vi "AWG Waveform Generator.vi"() -> ()   [LabVIEW 2020]
doc: "This example shows how to use the Arbitrary Waveform mode."
uses:
  <instrlib>/niFgen/niFgen.llb/niFgen Output Mode.ctl
  <instrlib>/niFgen/niFgen.llb/niFgen Trigger Mode.ctl
  <instrlib>/niFgen/niFgen.llb/niFgen Create Waveform (WDT).vi
panel:
  in  "Transient":T1={"t1 (ms)"=10.0, "t2 (ms)"=10.0, "t3 (ms)"=10.0, "High Load (A)"=1.0, "Low Load (A)"=0.0, "Slew rate A/us"=0.001}
  in  "error out":errorcluster
  out "Max Waveform size-Read":i32 format="%_1p"
  out "Waveform Graph":waveform(dbl)(graph)
  in  "Update":bool
  in  "DC Offset (V)":dbl(knob) scale=-0.5..0.5 scale format="%#.1f"
  in  "Gain":dbl(knob)=1.0 min=0.0 max=5.0 scale=0.0..10.0 scale format="%#.1f"
  in  "Stop":bool
  in  "FGEN Resource Name":refnum<k15>
  out "Actual Sample Rate (S/s)":dbl format="%.2p"
  in  "Sample Rate (S/s)":dbl=20000000.0 format="%.2p"
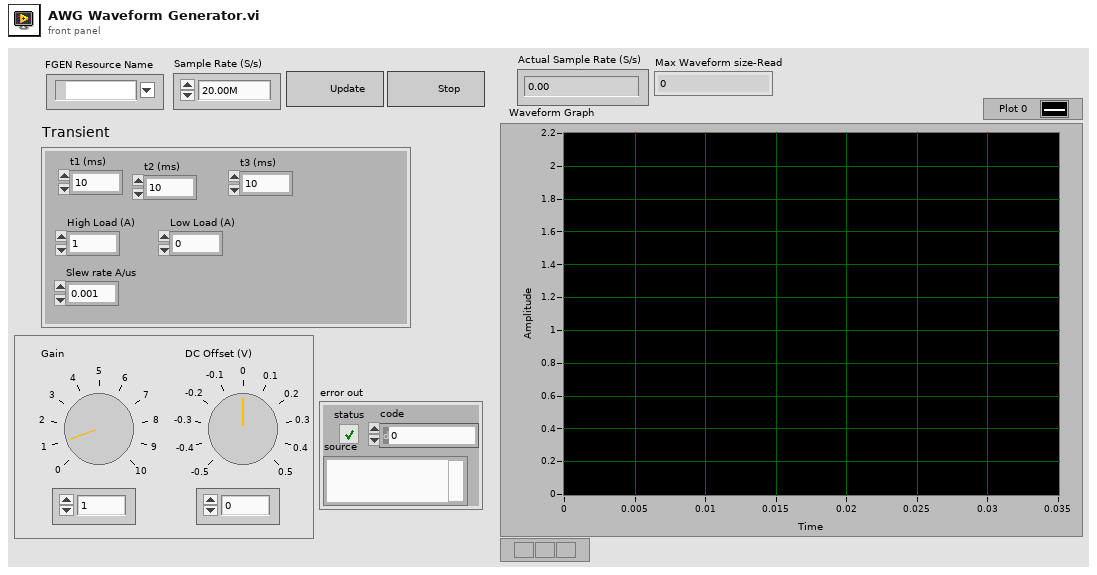
[diagram p1: front panel]
types:
  T1 = cluster{"t1 (ms)":dbl, "t2 (ms)":dbl, "t3 (ms)":dbl, "High Load (A)":dbl, "Low Load (A)":dbl, "Slew rate A/us":dbl}
  T2 = typedef "niFgen Trigger Mode.ctl" = i32
  T3 = typedef "niFgen Output Mode.ctl" = u32
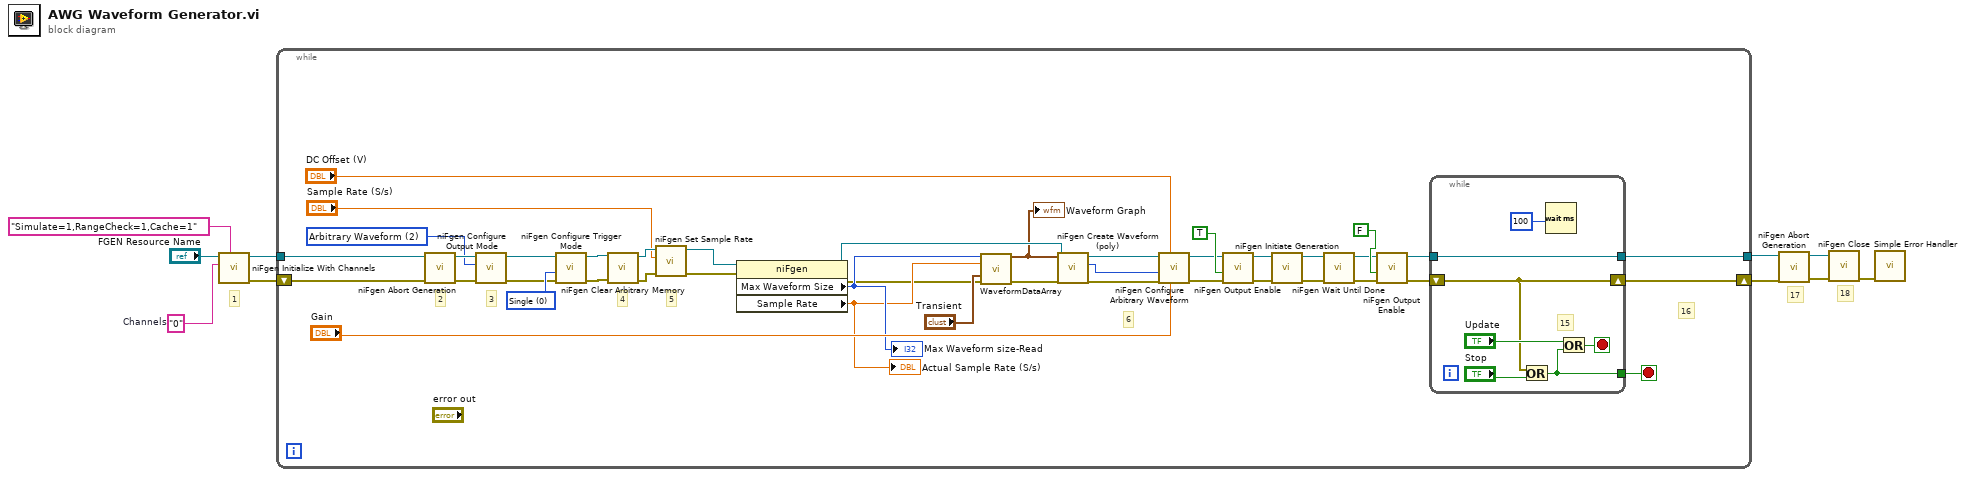
[diagram p0: block diagram]
diagram:
  w4 = "0"  # Channels
  # "18"
  # "17"
  # "1"
  n1 = call <instrlib>:"niFgen Initialize With Channels.vi"("Option String"="Simulate=1,RangeCheck=1,Cache=1", "Channel Name"=w4, "Resource Name"="FGEN Resource Name") -> ("error out"=w3:errorcluster, "Instrument Handle Out"=w2:refnum<k15>)  [unwired: 7 in]
  n2 = while {
    tunnel: [w11] -> w10
    tunnel: w2 -> [w51]
    shift-right: [w13] -> w6
    shift-left: w3 -> [w42]
    stop <- w39 stop-if-true
    w29 = T2 0 items=["Single", "Continuous", "Stepped", "Burst"] ("Trigger Mode")
    w44 = T3 2 items=["Standard Function", "Frequency List", "Arbitrary Waveform", "Arbitrary Sequence", "Script"] ("Output Mode")
    # "16"
    # "6"
    # "5"
    # "4"
    # "3"
    # "2"
    n3 = call <instrlib>:"niFgen Abort Generation.vi"("error in (no error)"=w42, "Instrument Handle"=w51) -> ("error out"=w48:errorcluster, "Instrument Handle Out"=w47:refnum<k15>)  [unwired: 8 in]
    n4 = call <instrlib>:"niFgen Configure Output Mode.vi"("error in (no error)"=w48, "Output Mode (default: 0=Standard Function)"=w44, "Instrument Handle"=w47) -> ("error out"=w27:errorcluster, "Instrument Handle Out"=w28:refnum<k15>)  [unwired: 6 in]
    n5 = call <instrlib>:"niFgen Configure Trigger Mode.vi"("error in (no error)"=w27, "Trigger Mode (default: 1=continuous)"=w29, "Instrument Handle"=w28) -> ("error out"=w25:errorcluster, "Instrument Handle Out"=w26:refnum<k15>)  [unwired: 7 in]
    n6 = call <instrlib>:"niFgen Clear Arbitrary Memory.vi"("error in (no error)"=w25, "Instrument Handle"=w26) -> ("error out"=w35:errorcluster, "Instrument Handle Out"=w36:refnum<k15>)  [unwired: 8 in]
    n7 = call <instrlib>:"niFgen Set Sample Rate.vi"("error in (no error)"=w35, "Sample Rate (Samp/s)"="Sample Rate (S/s)", "Instrument Handle"=w36) -> ("error out"=w30:errorcluster, "Instrument Handle Out"=w31:refnum<k15>)  [unwired: 7 in]
    n8 = property class="niFgen"(reference=w31, error in=w30) -> (reference out=w19:refnum<k15>, error out=w21:errorcluster, "Max Waveform Size"=w23:i32, "Sample Rate"=w22:dbl)
    "Actual Sample Rate (S/s)" <- w22
    "Max Waveform size-Read" <- w23
    n9 = call "WaveformDataArray.vi"("Max Waveform Size"=w23, "Sample Rate"=w22, "Transient"="Transient", "error in"=w21) -> ("Waveform Graph 2"=w18:waveform(dbl), "error out"=w20:errorcluster)  [unwired: 9 in, 1 out]
    "Waveform Graph" <- w18
    n10 = call-poly <instrlib>:"niFgen Create Waveform (poly).vi"("error in (no error)"=w20, "Waveform"=w18, "Instrument Handle"=w19) -> ("error out"=w49:errorcluster, "Waveform Handle"=w37:i32, "Instrument Handle Out"=w50:refnum<k15>)  [unwired: 6 in]
    n11 = call <instrlib>:"niFgen Configure Arbitrary Waveform.vi"("Gain"="Gain", "Offset"="DC Offset (V)", "error in (no error)"=w49, "Waveform Handle"=w37, "Instrument Handle"=w50) -> ("error out"=w32:errorcluster, "Instrument Handle Out"=w33:refnum<k15>)  [unwired: 5 in]
    n12 = call <instrlib>:"niFgen Output Enable.vi"("error in (no error)"=w32, "Output Enable (default: True)"=TRUE ("output enable"), "Instrument Handle"=w33) -> ("error out"=w45:errorcluster, "Instrument Handle Out"=w46:refnum<k15>)  [unwired: 7 in]
    n13 = call <instrlib>:"niFgen Initiate Generation.vi"("error in (no error)"=w45, "Instrument Handle"=w46) -> ("error out"=w16:errorcluster, "Instrument Handle Out"=w17:refnum<k15>)  [unwired: 8 in]
    n14 = call <instrlib>:"niFgen Wait Until Done.vi"("error in (no error)"=w16, "Instrument Handle"=w17) -> ("error out"=w14:errorcluster, "Instrument Handle Out"=w15:refnum<k15>)  [unwired: 8 in]
    n15 = call <instrlib>:"niFgen Output Enable.vi"("error in (no error)"=w14, "Output Enable (default: True)"=FALSE ("output enable"), "Instrument Handle"=w15) -> ("error out"=w13:errorcluster, "Instrument Handle Out"=w12:refnum<k15>)  [unwired: 7 in]
    n16 = while {
      tunnel: w12 -> [w53]
      tunnel: [w54] -> w39
      tunnel: [w53] -> w11
      shift-right: [w52] -> _
      shift-left: w13 -> [w52]
      stop <- w57 stop-if-true
      # "The case structure ensures that only valid values \nare used for DC Offset because the offset values \ndependent on the configured Gain Value."
      # "15"
      n17 = Or(x=w52, y="Stop") -> (x .or. y?=w54:bool)
      n18 = Wait (ms)(milliseconds to wait=u32 100 ("millisecond multiple")) -> ()  [unwired: 1 out]
      n19 = Or(x="Update", y=w54) -> (x .or. y?=w57:bool)
    }
  }
  n20 = call <instrlib>:"niFgen Abort Generation.vi"("error in (no error)"=w6, "Instrument Handle"=w10) -> ("error out"=w9:errorcluster, "Instrument Handle Out"=w8:refnum<k15>)  [unwired: 8 in]
  n21 = call <instrlib>:"niFgen Close.vi"("error in (no error)"=w9, "Instrument Handle"=w8) -> ("error out"=w7:errorcluster)  [unwired: 9 in]
  n22 = call <vilib>:"Simple Error Handler.vi"("error in (no error)"=w7) -> ()  [unwired: 4 in, 5 out]
